vi "Validate Channel.vi"(8 "error in":errorcluster, 11 "Module Configuration":refnum<class "Module Configuration.lvclass">) -> (0 "error out":errorcluster, 1 "Result Messages":T1[](array[typedef]), 2 "Config OK":bool, 3 "Module Configuration out":refnum<class "Module Configuration.lvclass">)   [LabVIEW 2020, in "Plugin.lvlib" / "Plugin_Controller.lvclass"]
doc: "Validates the channel for test execution"
uses:
  Plugin_Controller.lvclass
  builds/Libraries/LabSys Framework.lvlibp/Configuration Storage/Module Configuration/Module Configuration.lvclass
  builds/Libraries/LabSys Framework.lvlibp/Data Node/Data Node/Result.ctl
  builds/Libraries/LabSys Framework.lvlibp/Data Node/Data Node/Result Type.ctl
  UI_Class/Plugin_UI.lvclass
  builds/Libraries/LabSys Framework.lvlibp/Data Node/Data Node/Data Node.lvclass
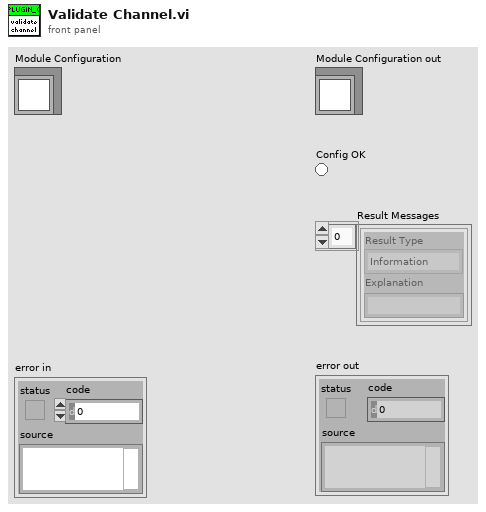
[diagram p1: front panel]
types:
  T1 = typedef "LabSys Framework.lvlibp/Data Node.lvlib/Data Node.lvclass/Result.ctl" = cluster{"Result Type":T2, "Explanation":string}
  T2 = typedef "LabSys Framework.lvlibp/Data Node.lvlib/Data Node.lvclass/Result Type.ctl" = enum16{"Information", "Warning", "Error"}
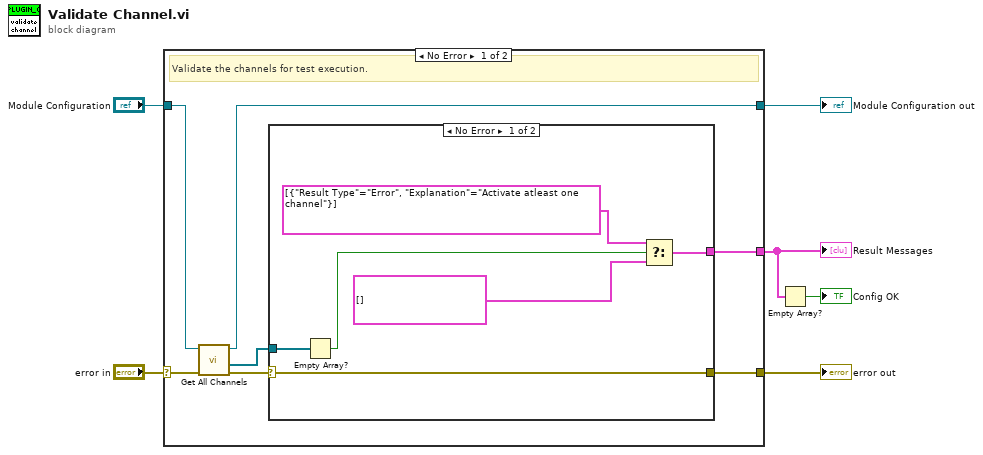
[diagram p0: block diagram]
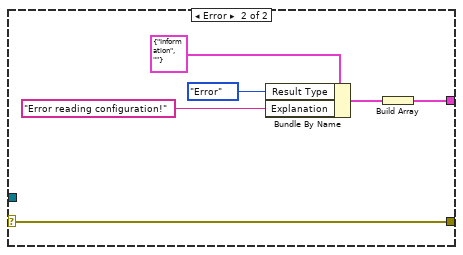
[diagram p2: hidden frame]
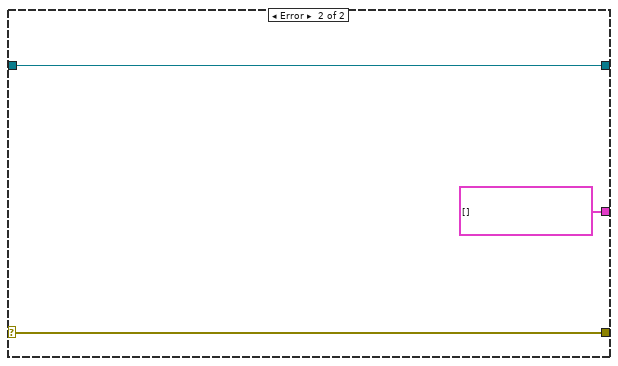
[diagram p3: hidden frame]
diagram:
  n1 = case shown="No Error" "error in" {
    selector: "error in" -> [w12 w28]
    tunnel: [w9 w28] -> w5
    tunnel: "Module Configuration" -> [w13 w26]
    tunnel: [w8 T1[] [] ("f")] -> w1
    tunnel: [w7 w26] -> w2
    frame No Error {
      # "Validate the channels for test execution."
      n2 = call "Get All Channels.vi"("error in (no error)"=w12, "Module Configuration"=w13) -> ("error out"=w11:errorcluster, "Output Channels[]"=w10:refnum<class "Output Channels.lvclass">[], "Module Configuration out"=w7:refnum<class "Module Configuration.lvclass">)  [unwired: 5 in, 2 out]
      n3 = case shown="No Error" w11 {
        selector: w11 -> [w15 w20]
        tunnel: w10 -> [w19 _]
        tunnel: [w15 w20] -> w9
        tunnel: [w14 w21] -> w8
        frame No Error {
          n4 = Empty Array?(array=w19) -> (empty?=w18:bool)
          n5 = Select(t=T1[] [{"Result Type"=enum."Error", "Explanation"="Activate atleast one channel"}], s=w18, f=T1[] []) -> (s? t:f=w14:T1[])
        }
        frame Error {
          n6 = Bundle By Name(cluster=T1 {"Result Type"=enum."Information", "Explanation"=""}, "Result Type"=Result_Type."Error", "Explanation"="Error reading configuration!") -> (w22:T1)
          n7 = Build Array(w22) -> (w21:T1[])
        }
      }
    }
    frame Error {
    }
  }
  "error out" <- w5
  "Module Configuration out" <- w2
  "Result Messages" <- w1
  n8 = Empty Array?(array=w1) -> (empty?=→"Config OK":bool)
